vi "test.vi"(11 "invalue":dbl) -> (0 "plain message":dbl, 3 "encrypted Out":dbl)   [LabVIEW 2024]
panel:
  in  "Python path":path
  in  "function name":string
  in  "module path":path
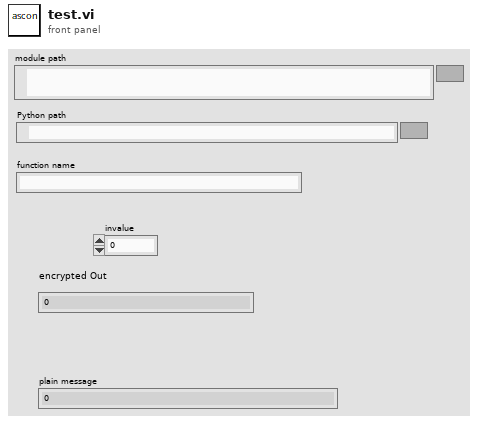
[diagram p1: front panel]
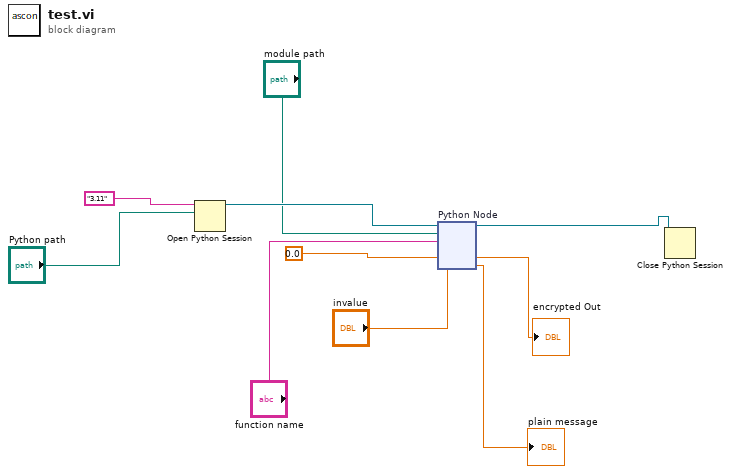
[diagram p0: block diagram]
diagram:
  n1 = Open Python Session(python version="3.11" ("Python version"), python path="Python path") -> (session out=w9:refnum<k35>)  [unwired: 1 in, 1 out]
  n2 = node "Python Node"(w9, "module path", "function name", 0.0, "invalue") -> (w3:refnum<k35>, →"encrypted Out":dbl, →"plain message":dbl)  [unwired: 1 in, 3 out]
  n3 = Close Python Session(session in=w3) -> ()  [unwired: 1 in, 1 out]
